vi "formatIntoRowInterface.vi"(8 "error in (no error)":errorcluster, 11 "Goal in":refnum<class "Goal.lvclass">) -> (0 "error out":errorcluster, 2 "Row Interface":string[](array[string]), 3 "Goal out":refnum<class "Goal.lvclass">)   [LabVIEW 2018, in "Goal.lvclass"]
uses:
  Goal.lvclass
  C:/GitRepos/Filthy-Lucre-Budgetizer/source/support/classes/UserEditableAmount/UserEditableAmount.lvclass
  Goal.lvclass/Goal.ctl
  Category/Category.lvclass
  UserEditableAmount/UserEditableAmount.lvclass
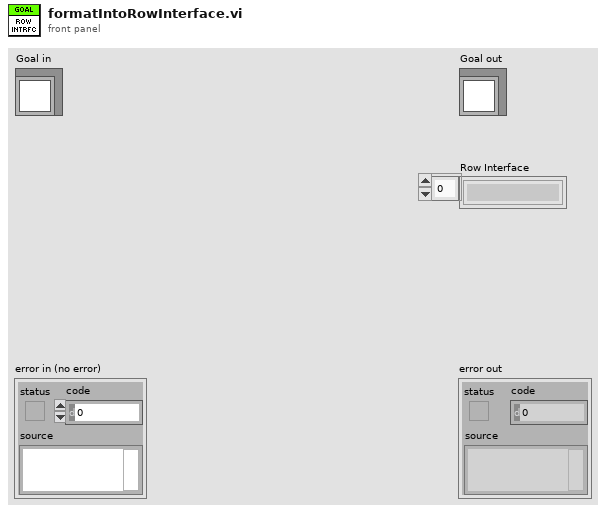
[diagram p1: front panel]
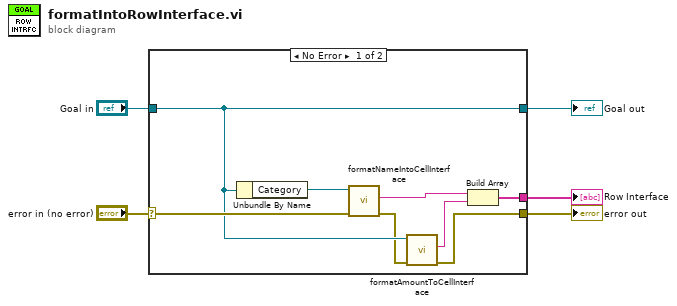
[diagram p0: block diagram]
diagram:
  n1 = case shown="No Error" "error in (no error)" {
    selector: "error in (no error)" -> [w12 w15]
    tunnel: [w7 w15] -> w4
    tunnel: [w11 w14] -> w2
    tunnel: "Goal in" -> [w11 w14]
    tunnel: [w6 _] -> w1
    frame No Error {
      n2 = Unbundle By Name(w11) -> ("Category"=w13:refnum<class "Category.lvclass">)
      n3 = call "formatNameIntoCellInterface.vi"("error in (no error)"=w12, "Category in"=w13) -> ("error out"=w10:errorcluster, "Name"=w9:string)  [unwired: 7 in, 1 out]
      n4 = call "formatAmountToCellInterface.vi"("error in (no error)"=w10, "UserEditableAmount in"=w11) -> ("error out"=w7:errorcluster, "Cell Interface"=w8:string)  [unwired: 7 in, 1 out]
      n5 = Build Array(w9, w8) -> (w6:string[])
    }
    frame Error {
    }
  }
  "error out" <- w4
  "Goal out" <- w2
  "Row Interface" <- w1
